vi "Configure Averaging.vi"(6 "Block Size (15)":i32=15, 8 "error in (no error)":errorcluster, 9 "Number of readings (0:4)":i32(ring) items=["4", "16", "64"], 10 "Mode (0: Rolling Average)":u16(ring) items=["Rolling Average", "Block Average", "OFF"], 11 "VISA resource name":refnum<visa-resource-name>) -> (0 "error out":errorcluster, 3 "VISA resource name out":refnum<visa-resource-name>)   [LabVIEW 2011, in "Fluke 8508.lvlib"]
doc: "This VI sets the averaging function on the instrument and configures the various averaging parameters.\n\nCombinations of math VIs are allowed, but they must be performed in the following order:\n1. Averaging\n2. Multiplication \n3. Subtraction \n4. Division\n5. Decibels"
uses:
  Fluke 8508.lvlib
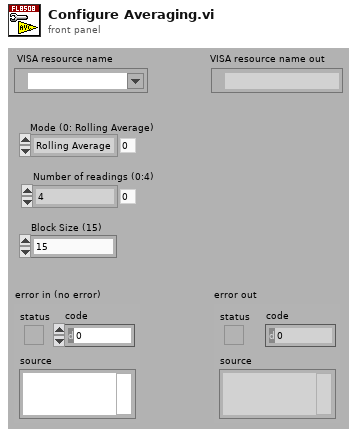
[diagram p1: front panel]
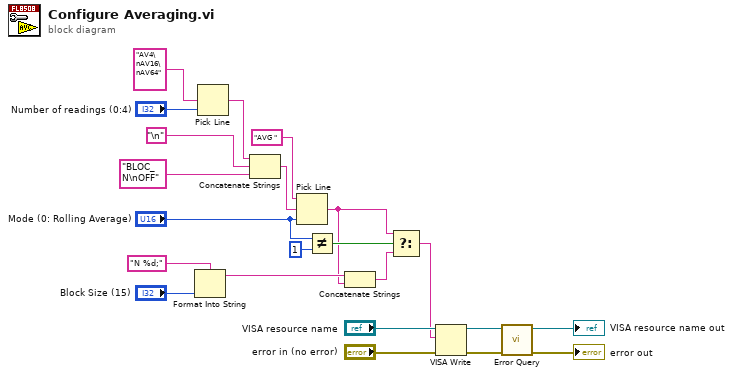
[diagram p0: block diagram]
diagram:
  n1 = Format Into String(format string="N %d;", "Block Size (15)") -> (resulting string=w11:string)  [unwired: 2 in, 1 out]
  n2 = Pick Line(multi-line string="AV4\nAV16\nAV64", line index="Number of readings (0:4)") -> (output string=w7:string)  [unwired: 1 in]
  n3 = Concatenate Strings(w7, "\n" ("format string"), "BLOC_N\nOFF" ("string")) -> (w8:string)
  n4 = Pick Line(string ("")="AVG ", multi-line string=w8, line index="Mode (0: Rolling Average)") -> (output string=w10:string)
  n5 = Not Equal?(x="Mode (0: Rolling Average)", y=u16 1) -> (x != y?=w14:bool)
  n6 = Concatenate Strings(w11, w10) -> (w13:string)
  n7 = Select(t=w10, s=w14, f=w13) -> (s? t:f=w12:string)
  n8 = VISA Write(VISA resource name="VISA resource name", write buffer=w12, error in (no error)="error in (no error)") -> (VISA resource name out=w3:refnum<visa-resource-name>, error out=w5:errorcluster)  [unwired: 1 out]
  n9 = call "Error Query.vi"("error in (no error)"=w5, "VISA resource name"=w3) -> ("error out"=→"error out":errorcluster, "VISA resource name out"=→"VISA resource name out":refnum<visa-resource-name>)  [unwired: 6 in, 2 out]
